vi "About.vi"() -> ()   [LabVIEW 2016]
panel:
  out "Version":string
  out "Authors":string
  in  "App_Name":string="Eye Movement Analyzer"
  # "Copyright (c) 2014 NeuRA - Balance and Vision Lab.\nAll rights reserved by Authors"
  # "Authors"
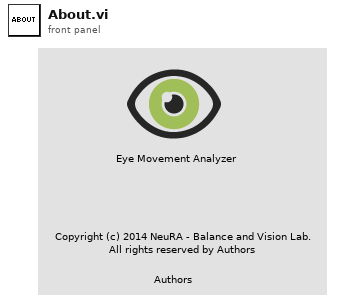
[diagram p1: front panel]
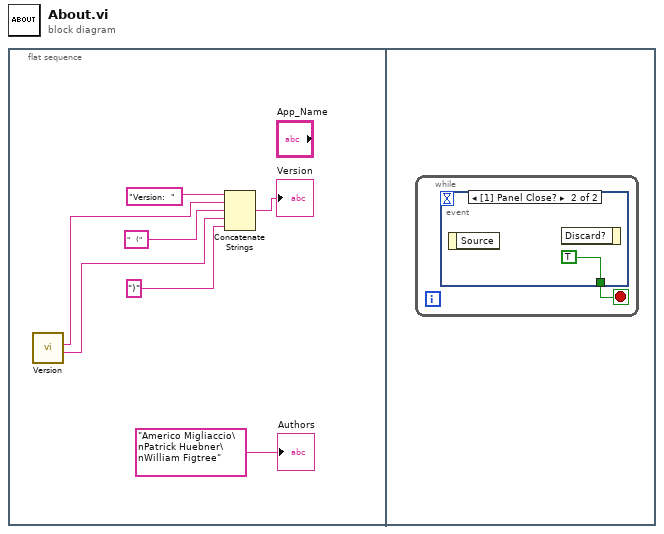
[diagram p0: block diagram]
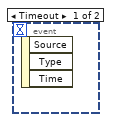
[diagram p2: hidden frame]
diagram:
  n1 = flat-sequence {
    frame #0 {
      n2 = call "Version.vi"() -> ("Build"=w1:string, "Version"=w2:string)  [unwired: 10 in]
      n3 = Concatenate Strings("Version:  ", w2, "   (", w1, ")" ("string")) -> (→"Version":string)
      "Authors" <- "Americo Migliaccio\nPatrick Huebner\nWilliam Figtree"
    }
    frame #1 {
      n4 = while {
        stop <- w8 stop-if-true
        n5 = event shown="[1] Panel Close?" {
          selector: _ -> [_ _]
          dyn-events: _ -> [_ _]
          timeout: _ -> [_ _]
          tunnel: [_ TRUE] -> w8
          event Timeout {
            n6 = event-data() -> ()  [unwired: 1 in, 3 out]
          }
          event Panel Close? {
            n7 = event-data() -> ()  [unwired: 1 in, 1 out]
            n8 = event-data() -> ()  [unwired: 2 in, 1 out]
          }
        }
      }
    }
  }
